vi "PopSubpanelHandler.vi"(8 "error in (no error)":errorcluster, 10 "EmbeddedSMO in":refnum<class "SMO.UI.Embedded.lvclass">, 11 "SMO.UI.MAUI in":refnum<class "SMO.UI.MAUI.lvclass">) -> (0 "error out":errorcluster, 3 "SMO.UI.MAUI out":refnum<class "SMO.UI.MAUI.lvclass">)   [LabVIEW 2016, in "SMO.UI.MAUI.lvclass"]
uses:
  SMO.UI.MAUI.lvclass
  <vilib>/Levylab/SMO.UI.Embedded/SMO.UI.Embedded.lvclass
  C:/Program Files (x86)/National Instruments/LabVIEW 2016/vi.lib/JKI/JKI SMO/SMO/SMO.lvclass
  SMO.UI.MAUI.lvclass/SMO.UI.MAUI.ctl
  <vilib>/JKI/JKI SMO/SMO/SMO.lvclass
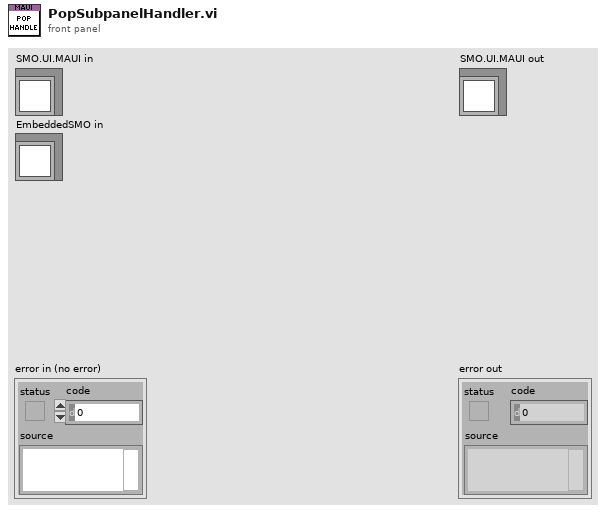
[diagram p1: front panel]
types:
  T1 = typedef "SMO.UI.MAUI.lvclass/PanelData.ctl" = cluster{"SubPanel":refnum<vi>, "Ring":refnum<vi>, "Active":i32}
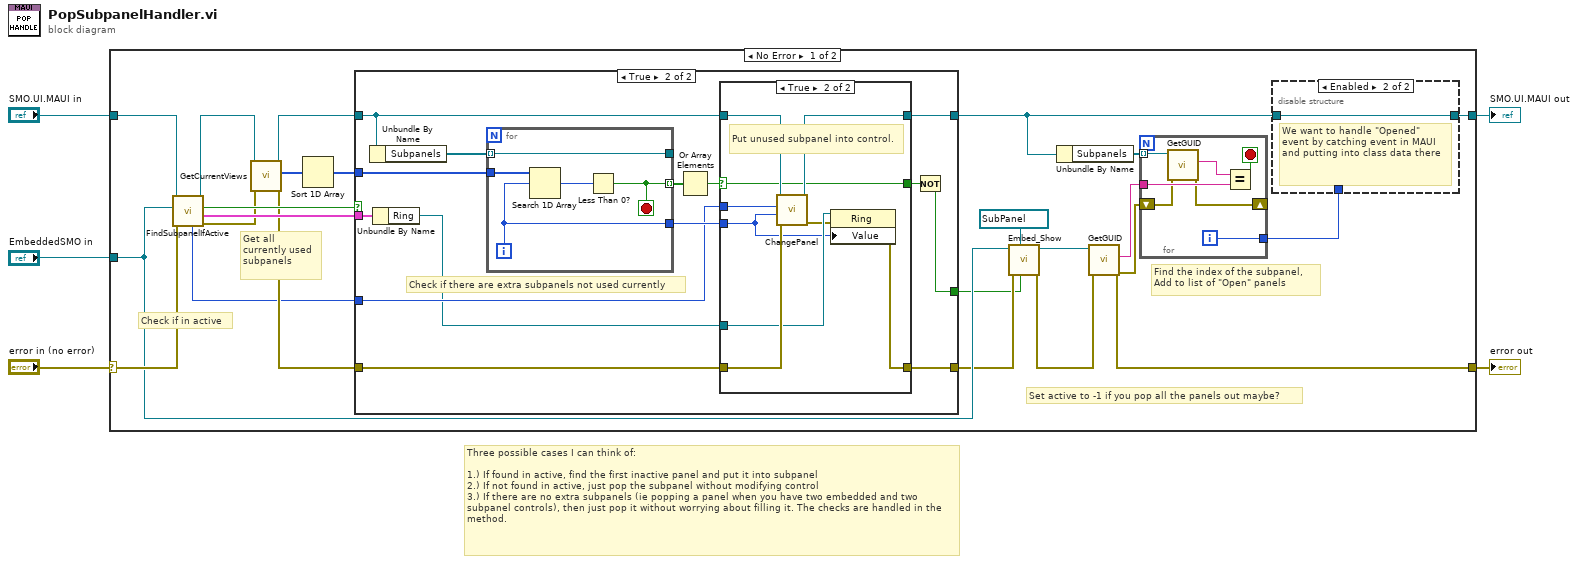
[diagram p0: block diagram]
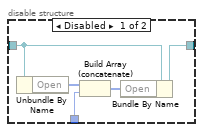
[diagram p2: hidden frame]
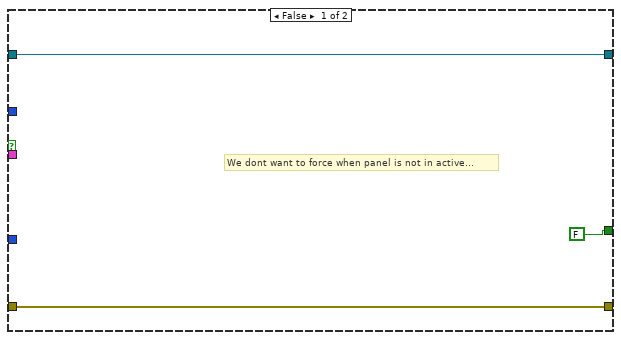
[diagram p3: hidden frame]
diagram:
  # "Three possible cases I can think of:\n\n1.) If found in active, find the first inactive panel and put it into subpanel\n2.) If not found in active, just pop the subpanel without modifying control\n3.) If there are no extra subpanels (ie popping a panel when you have two embedded and two subpanel controls), then just pop it without worrying about filling it. The checks are handled in the method."
  n1 = case shown="No Error" "error in (no error)" {
    selector: "error in (no error)" -> [w27 w77]
    tunnel: [w10 w77] -> w4
    tunnel: [w9 w76] -> w2
    tunnel: "SMO.UI.MAUI in" -> [w28 w76]
    tunnel: "EmbeddedSMO in" -> [w17 _]
    frame No Error {
      # "Set active to -1 if you pop all the panels out maybe?"
      # "Find the index of the subpanel, \nAdd to list of \"Open\" panels"
      # "Check if in active"
      # "Get all currently used subpanels"
      n2 = call "FindSubpanelIfActive.vi"("error in (no error)"=w27, "EmbeddedSMO in"=w17, "SMO.UI.MAUI in"=w28) -> ("error out"=w22:errorcluster, "Panel"=w25:T1, "Found?"=w26:bool, "SMO.UI.MAUI out"=w24:refnum<class "SMO.UI.MAUI.lvclass">, "Panel Index"=w18:i32)  [unwired: 4 in]
      n3 = call "GetCurrentViews.vi"("error in (no error)"=w22, "SMO.UI.MAUI in"=w24) -> ("error out"=w21:errorcluster, "Current Views"=w20:i32[], "SMO.UI.MAUI out"=w23:refnum<class "SMO.UI.MAUI.lvclass">)  [unwired: 7 in]
      n4 = Sort 1D Array(array=w20) -> (sorted array=w19:i32[])
      n5 = case shown="True" w26 {
        tunnel: w25 -> [_ w48]
        tunnel: w21 -> [w44 w50]
        tunnel: [w44 w49] -> w16
        tunnel: w23 -> [w43 w52]
        tunnel: [w43 w51] -> w8
        tunnel: w19 -> [_ w57]
        tunnel: w18 -> [_ w53]
        tunnel: [FALSE w45] -> w6
        frame False {
          # "We dont want to force when panel is not in active..."
        }
        frame True {
          # "Check if there are extra subpanels not used currently"
          n6 = Unbundle By Name(w52) -> ("Subpanels"=w58:refnum<class "SMO.UI.Embedded.lvclass">[])
          n7 = Unbundle By Name(w48) -> ("Ring"=w47:refnum<vi>)
          n8 = for {
            tunnel: w58 -> [w73] mode=indexing
            tunnel: w57 -> [w75]
            tunnel: [w73] -> _
            tunnel: [w72] -> w56 mode=indexing
            tunnel: [w71] -> w54
            i -> [w71]
            stop <- w72 stop-if-true
            n9 = Search 1D Array(1D array=w75, element=w71) -> (index of element=w74:i32)  [unwired: 1 in]
            n10 = Less Than 0?(x=w74) -> (x < 0?=w72:bool)
          }
          n11 = Or Array Elements(Boolean array=w56) -> (logical OR=w55:bool)
          n12 = case shown="True" w55 {
            selector: w55 -> [w59 w65]
            tunnel: w52 -> [w61 w70]
            tunnel: w54 -> [_ w64]
            tunnel: w53 -> [_ w69]
            tunnel: [w61 w68] -> w51
            tunnel: w50 -> [w60 w67]
            tunnel: [w60 w62] -> w49
            tunnel: w47 -> [_ w66]
            tunnel: [w59 w65] -> w46
            frame False {
              # "We want to force a pop when there is no more extra subpanels."
            }
            frame True {
              # "Put unused subpanel into control."
              n13 = call "ChangePanel.vi"("error in (no error)"=w67, "New Active Index"=w64, "Panel Index"=w69, "MAUI in"=w70) -> ("error out"=w63:errorcluster, "MAUI out"=w68:refnum<class "SMO.UI.MAUI.lvclass">)  [unwired: 6 in]
              n14 = property class="Ring"(reference=w66, error in=w63, "Value"=w64) -> (error out=w62:errorcluster)  [unwired: 1 out]
            }
          }
          n15 = Not(x=w46) -> (.not. x?=w45:bool)
        }
      }
      n16 = call <vilib>:"Embed_Show.vi"("Force?"=w6, "Sub Panel"=refnum<vi> refnum, "error in (no error)"=w16, "EmbeddedSMO in"=w17) -> ("error out"=w12:errorcluster, "EmbeddedSMO out"=w13:refnum<class "SMO.UI.Embedded.lvclass">)  [unwired: 6 in]
      n17 = Unbundle By Name(w8) -> ("Subpanels"=w14:refnum<class "SMO.UI.Embedded.lvclass">[])
      n18 = call <vilib>:"GetGUID.vi"("error in (no error)"=w12, "SMO"=w13) -> ("error out"=w10:errorcluster, "GUID"=w11:string)  [unwired: 7 in, 1 out]
      n19 = for {
        tunnel: w14 -> [w41] mode=indexing
        tunnel: w11 -> [w39]
        tunnel: [w37] -> w7
        shift-right: [w35] -> _
        shift-left: w10 -> [w36]
        i -> [w37]
        stop <- w38 stop-if-true
        n20 = call <vilib>:"GetGUID.vi"("error in (no error)"=w36, "SMO"=w41) -> ("error out"=w35:errorcluster, "GUID"=w40:string)  [unwired: 7 in, 1 out]
        n21 = Equal?(x=w40, y=w39) -> (x = y?=w38:bool)
      }
      n22 = disable-structure shown="Enabled" {
        disable-tunnel: [w33 w34] -> w9
        disable-tunnel: w8 -> [w32 w34]
        disable-tunnel: w7 -> [w29 _]
        frame Disabled {
          n23 = Unbundle By Name(w32) -> ("Open"=w31:i32[])
          n24 = Build Array (concatenate)(w31, w29) -> (w30:i32[])
          n25 = Bundle By Name(cluster=w32, "Open"=w30) -> (w33:refnum<class "SMO.UI.MAUI.lvclass">)
        }
        frame Enabled {
          # "We want to handle \"Opened\" event by catching event in MAUI and putting into class data there"
        }
      }
    }
    frame Error {
    }
  }
  "error out" <- w4
  "SMO.UI.MAUI out" <- w2
